vi "Read Write Profile.vi"(4 "Channel to Read":T2, 7 "Refresh":bool, 9 "Channel to Write":T2, 10 "Channel List In":T3[](array[typedef])) -> (0 "Bitfile Read?":bool, 2 "Channel List Out":T3[](array[typedef]), 3 "Profile Data Out":T1[](array[typedef]))   [LabVIEW 2021]
uses:
  <vilib>/myRIO/Common/Profile Manager Framework/typedefs/Channel Type Profile.ctl
  <vilib>/myRIO/Common/Instrument Driver Framework/Utilities/typedefs/Channel Types.ctl
  <vilib>/myRIO/Common/Profile Manager Framework/typedefs/Channel Info.ctl
panel:
  in  "Channel Type Profile In":T1
  out "Channel Type Profile Out":T1
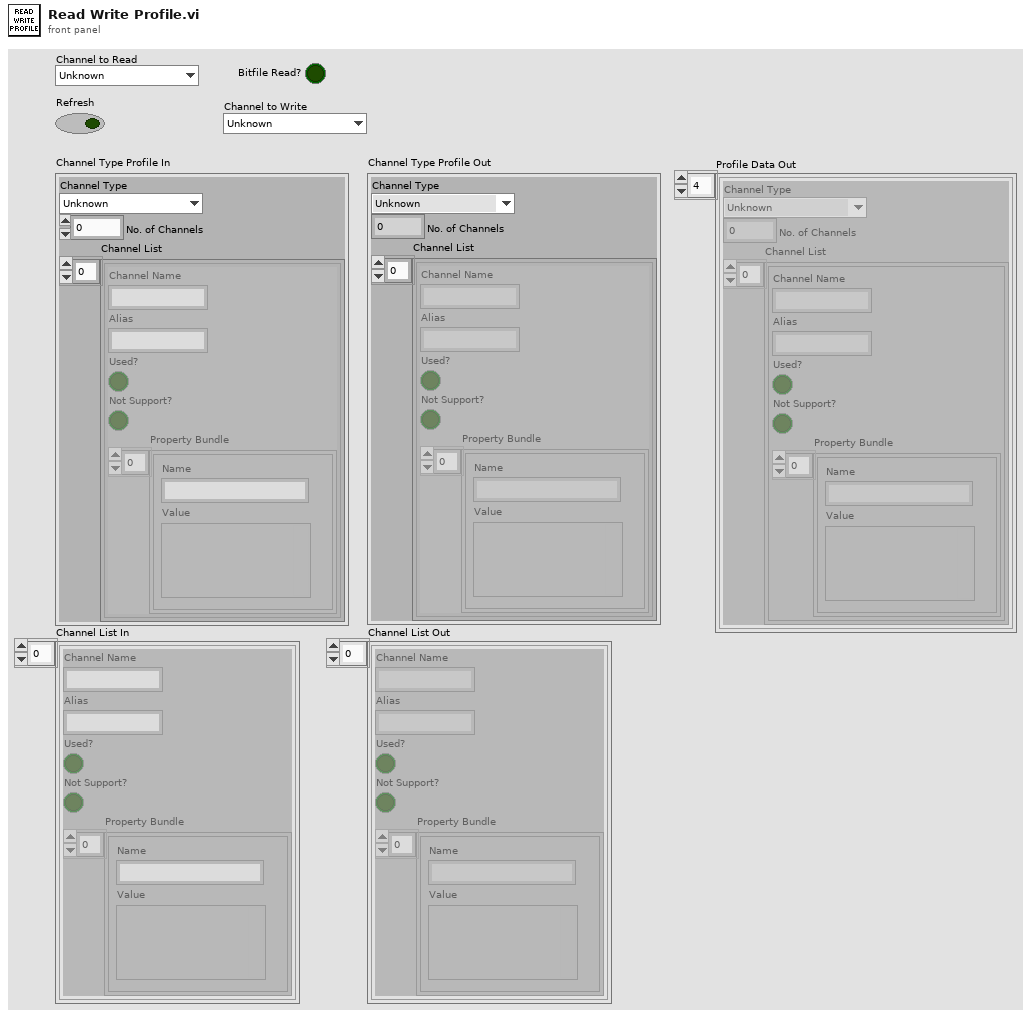
[diagram p1: front panel]
types:
  T1 = typedef "Channel Type Profile.ctl" = cluster{"Channel Type":T2, "No. of Channels":dbl, "Channel List":T3[]}
  T2 = typedef "Channel Types.ctl" = enum32{"Unknown", "AI", "AO", "DIO - DI", "DIO", "DIO - DO", "I2C", "PWM", "Encoder", "SPI", "UART", "Accelerometer", "DIO - LED", "DIO - Button", "AI (N Samples)", "AudioIn (N Samples)", "AO (N Samples)", "AudioOut (N Samples)", "DI (N Samples)", "DO (N Samples)", "AI IRQ", "DI IRQ", "Timer IRQ", "RSL", "Relay", "CAN", "AI (Continuous)", "AO (Continuous)"}
  T3 = typedef "Channel Info.ctl" = cluster{"Channel Name":string, "Alias":string, "Used?":bool, "Not Support?":bool, "Property Bundle":cluster{"Name":string, "Value":variant}[]}
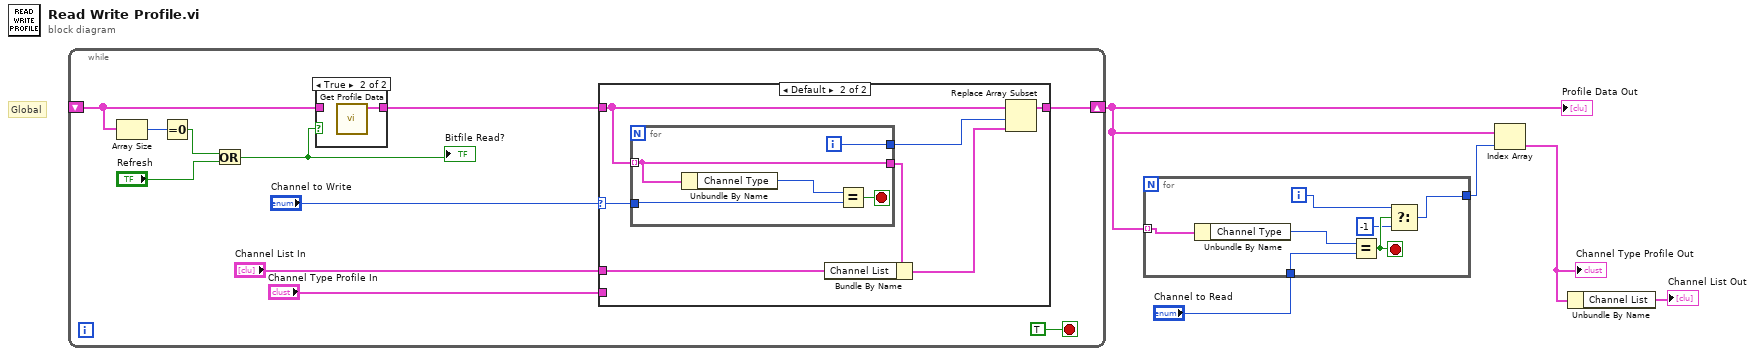
[diagram p0: block diagram]
diagram:
  # "Global"
  n1 = while {
    shift-right: [w14] -> w1
    shift-left: _ -> [w12]
    stop <- TRUE stop-if-true
    n2 = Array Size(array=w12) -> (size(s)=w11:i32)
    n3 = Equal To 0?(x=w11) -> (x = 0?=w10:bool)
    n4 = Or(x=w10, y="Refresh") -> (x .or. y?=w8:bool)
    "Bitfile Read?" <- w8
    n5 = case shown="True" w8 {
      tunnel: [w30 w31] -> w15
      tunnel: w12 -> [w30 _]
      frame False {
      }
      frame True {
        n6 = call <vilib>:"Get Profile Data.vi"() -> ("Profile Data Out"=w31:T1[])  [unwired: 10 in, 1 out]
      }
    }
    n7 = case shown="Default" "Channel to Write" {
      selector: "Channel to Write" -> [_ w21]
      tunnel: w15 -> [w17 w24]
      tunnel: [w17 w23] -> w14
      tunnel: "Channel Type Profile In" -> [_ _]
      tunnel: "Channel List In" -> [_ w18]
      frame "Unknown" {
      }
      frame Default {
        n8 = for {
          tunnel: w24 -> [w25] mode=indexing
          tunnel: w21 -> [w28]
          tunnel: [w26] -> w22
          tunnel: [w25] -> w20
          i -> [w26]
          stop <- w27 stop-if-true
          n9 = Unbundle By Name(w25) -> ("Channel Type"=w29:T2)
          n10 = Equal?(x=w29, y=w28) -> (x = y?=w27:bool)
        }
        n11 = Bundle By Name(cluster=w20, "Channel List"=w18) -> (w19:T1)
        n12 = Replace Array Subset(array=w24, new element=w19, index=w22) -> (w23:T1[])
      }
    }
  }
  "Profile Data Out" <- w1
  n13 = for {
    tunnel: w1 -> [w38] mode=indexing
    tunnel: "Channel to Read" -> [w36]
    tunnel: [w34] -> w4
    i -> [w33]
    stop <- w35 stop-if-true
    n14 = Unbundle By Name(w38) -> ("Channel Type"=w37:T2)
    n15 = Equal?(x=w37, y=w36) -> (x = y?=w35:bool)
    n16 = Select(t=w33, s=w35, f=-1) -> (s? t:f=w34:i32)
  }
  n17 = Index Array(array=w1, index=w4) -> (element=w3:T1)
  "Channel Type Profile Out" <- w3
  n18 = Unbundle By Name(w3) -> ("Channel List"=→"Channel List Out":T3[])
